vi "TOOLweb EINSTELLUNGEN.vi"(4 "error in (no error)":errorcluster caption="Fehler (Eingang, kein Fehler)", 5 "IP-Adresse (localhost)":string="127.0.0.1") -> (3 "Einstellungen":T1)   [LabVIEW 2020, in "FT-IR.lvlib" / "TOOLweb Interface.lvlib"]
doc: "Holt mit einer HTTP-POST-Anforderung gemäß TOOLweb-Protokoll Einstellungen und Diagnose-Information vom MKS MultiGas 2030 Analyzer. Alle Daten werden zeitsparend in einem einzigen Poll Request zusammengefasst, damit nur einmal eine TCP/IP-Verbindung geöffnet werden muss.\n\nAlle Ergebnis-Datentypen sind als Typdefinitionen in der Bibliothek \"Datentypen\" enthalten\" und erlauben so eine spätere Erweiterung.\n\nFalls \"Anzahl Gase\" unverbunden bleibt, wird der Standardwert 18 verwendet.\n \nFalls der TOOLWeb-Server nicht auf demselben Rechner arbeitet, kann mit \"IP-Adresse\" eine beliebiger Host adressiert werden. Ein unverbundener Eingang spricht den lokalen Host an."
uses:
  TOOLweb Interface.lvlib
  TOOLweb Einstellungen.ctl
  Stoerungen/Stoerungen Messgeraet/Aktionen Kommunikation Stoerung.ctl
  TOOLweb Interface Hilfs-VIs.lvlib
  Typdefinitionen.lvlib
  Stoerungen/Stoerungen.lvlib
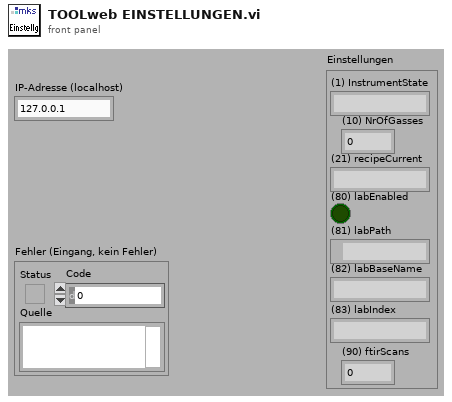
[diagram p1: front panel]
types:
  T1 = typedef "FT-IR.lvlib/TOOLweb Interface.lvlib/Typdefinitionen.lvlib/TOOLweb Einstellungen.ctl" = cluster{"(1) InstrumentState":string, "(10) NrOfGasses":i32, "(21) recipeCurrent":string, "(80) labEnabled":bool, "(81) labPath":path, "(82) labBaseName":string, "(83) labIndex":string, "(90) ftirScans":i32}
  T2 = typedef "Stoerungen.lvlib/Aktionen Kommunikation Stoerung.ctl" = enum16{"lesen", "init", "FT-IR Komm", "FT-IR Betriebsart", "FT-IR Hintergrund", "cRIO Komm", "PNS Komm", "Dichtheitstest", "Life Bit", "FTIR Komm AK", "PMA Komm", "FID Komm", "PMA Cal", "FID Ch4 Cal", "FID THC Cal", "Cal Timeout", "VFS 1 Komm", "VFS 2 Komm", "VFS 3 Komm", "VFS 4 Komm", "TRE 08 Komm", "CG-Test vorzeitig", "CG-Test Span 1", "CG-Test Span 2", "CG-Test Span 3", "CG-Test Messgas", "CG-Test löschen", "Test", "Amium AK", "AK Recept konfig", "AK Name konfig", "AK EKFG konfig"}
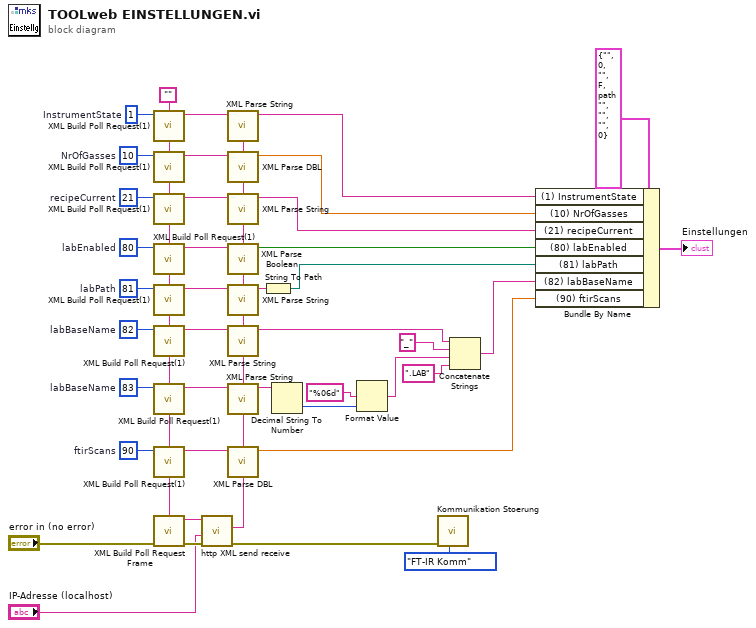
[diagram p0: block diagram]
diagram:
  w15 = 83  # labBaseName
  w35 = 90  # ftirScans
  w38 = 82  # labBaseName
  w44 = 81  # labPath
  w49 = 1  # InstrumentState
  w53 = 80  # labEnabled
  w54 = 21  # recipeCurrent
  w55 = 10  # NrOfGasses
  n1 = call "XML Build Poll Request(1).vi"("XML-Message alt"="", "EVID-Nummer"=w49) -> ("Attribut Name"=w48:string, "XML-Message neu"=w30:string)  [unwired: 6 out]
  n2 = call "XML Build Poll Request(1).vi"("XML-Message alt"=w30, "EVID-Nummer"=w55) -> ("Attribut Name"=w56:string, "XML-Message neu"=w22:string)  [unwired: 6 out]
  n3 = call "XML Build Poll Request(1).vi"("XML-Message alt"=w22, "EVID-Nummer"=w54) -> ("Attribut Name"=w52:string, "XML-Message neu"=w25:string)  [unwired: 6 out]
  n4 = call "XML Build Poll Request(1).vi"("XML-Message alt"=w25, "EVID-Nummer"=w53) -> ("Attribut Name"=w45:string, "XML-Message neu"=w32:string)  [unwired: 6 out]
  n5 = call "XML Build Poll Request(1).vi"("XML-Message alt"=w32, "EVID-Nummer"=w44) -> ("Attribut Name"=w42:string, "XML-Message neu"=w39:string)  [unwired: 6 out]
  n6 = call "XML Build Poll Request(1).vi"("XML-Message alt"=w39, "EVID-Nummer"=w38) -> ("Attribut Name"=w36:string, "XML-Message neu"=w13:string)  [unwired: 6 out]
  n7 = call "XML Build Poll Request(1).vi"("XML-Message alt"=w13, "EVID-Nummer"=w15) -> ("Attribut Name"=w16:string, "XML-Message neu"=w12:string)  [unwired: 6 out]
  n8 = call "XML Build Poll Request(1).vi"("XML-Message alt"=w12, "EVID-Nummer"=w35) -> ("Attribut Name"=w34:string, "XML-Message neu"=w11:string)  [unwired: 6 out]
  n9 = call "XML Build Poll Request Frame.vi"("XML-Message"=w11, "error in (no error)"="error in (no error)") -> ("XML-Message fertig"=w29:string, "error out"=w51:errorcluster)  [unwired: 1 in, 5 out]
  n10 = call "http XML send receive.vi"("error in (no error)"=w51, "IP-Adresse (localhost)"="IP-Adresse (localhost)", "XML Request"=w29) -> ("error out"=w17:errorcluster, "Response Body (XML)"=w14:string)  [unwired: 3 out]
  n11 = call "XML Parse DBL.vi"("Attribut Name"=w34, "XML Response"=w14) -> ("Wert (DBL)"=w33:dbl, "XML Response gekürzt"=w10:string)  [unwired: 6 out]
  n12 = call "XML Parse String.vi"("Attribut Name"=w16, "XML Response"=w10) -> ("Wert-String"=w6:string, "XML Response gekürzt"=w9:string)  [unwired: 6 out]
  n13 = call "XML Parse String.vi"("Attribut Name"=w36, "XML Response"=w9) -> ("Wert-String"=w5:string, "XML Response gekürzt"=w37:string)  [unwired: 6 out]
  n14 = call "XML Parse String.vi"("Attribut Name"=w42, "XML Response"=w37) -> ("Wert-String"=w41:string, "XML Response gekürzt"=w43:string)  [unwired: 6 out]
  n15 = call "XML Parse Boolean.vi"("Attribut Name"=w45, "XML Response"=w43) -> ("Wert (boolean)"=w28:bool, "XML Response gekürzt"=w24:string)  [unwired: 6 out]
  n16 = call "XML Parse String.vi"("Attribut Name"=w52, "XML Response"=w24) -> ("Wert-String"=w26:string, "XML Response gekürzt"=w21:string)  [unwired: 6 out]
  n17 = call "XML Parse DBL.vi"("Attribut Name"=w56, "XML Response"=w21) -> ("Wert (DBL)"=w46:dbl, "XML Response gekürzt"=w31:string)  [unwired: 6 out]
  n18 = call "XML Parse String.vi"("Attribut Name"=w48, "XML Response"=w31) -> ("Wert-String"=w47:string)  [unwired: 7 out]
  n19 = String To Path(string=w41) -> (path=w40:path)
  n20 = Decimal String To Number(string=w6) -> (number=w7:i32)  [unwired: 2 in, 1 out]
  n21 = Format Value(format string="%06d" ("Format-String"), value (0)=w7) -> (output string=w4:string)  [unwired: 1 in]
  n22 = call "Kommunikation Stoerung.vi"("Aktionen"=Aktionen_Kommunikation_Stoerung."FT-IR Komm", "error in"=w17) -> ()  [unwired: 9 in, 1 out]
  n23 = Concatenate Strings(w5, "_" ("String"), w4, ".LAB" ("String")) -> (w1:string)
  n24 = Bundle By Name(cluster=T1 {"(1) InstrumentState"="", "(10) NrOfGasses"=0, "(21) recipeCurrent"="", "(80) labEnabled"=FALSE, "(81) labPath"=path "", "(82) labBaseName"="", "(83) labIndex"="", "(90) ftirScans"=0} ("Info"), "(1) InstrumentState"=w47, "(10) NrOfGasses"=w46, "(21) recipeCurrent"=w26, "(80) labEnabled"=w28, "(81) labPath"=w40, "(82) labBaseName"=w1, "(90) ftirScans"=w33) -> (→"Einstellungen":T1)
